vi "CAN Task.vi"(8 "error in":errorcluster, 11 "CANopen Master in":refnum<class "CANopen Master.lvclass">) -> ()   [LabVIEW 2024, in "CANopen Master.lvlib" / "CANopen Master.lvclass"]
uses:
  CANopen Master.lvclass/CANopen Master.ctl
  CANopen Master.lvclass
  CANopen Message/CANopen Message.lvclass
  CANopen Response/CANopen Response Message.lvclass
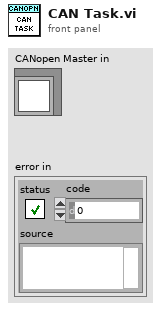
[diagram p1: front panel]
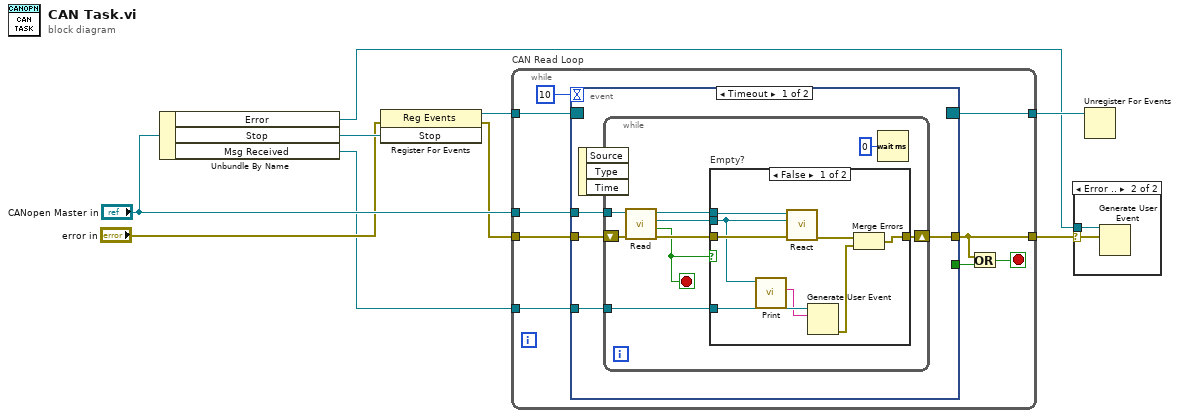
[diagram p0: block diagram]
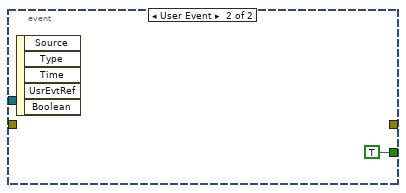
[diagram p4: hidden frame]
diagram:
  n1 = Unbundle By Name("CANopen Master in") -> ("Error"=w1:refnum<user-event>, "Stop"=w6:refnum<user-event>, "Msg Received"=w3:refnum<user-event>)
  n2 = register-events(error in="error in", w6) -> (reference out=w7:refnum<event-registration>, error out=w4:errorcluster)  [unwired: 1 in]
  n3 = while "CAN Read Loop" {
    tunnel: [w14] -> w9
    tunnel: w7 -> [w13]
    tunnel: w3 -> [w11]
    tunnel: "CANopen Master in" -> [w17]
    tunnel: w4 -> [w18]
    tunnel: [w10] -> w2
    stop <- w16 stop-if-true
    n4 = event shown="[0] Timeout" {
      selector: w13 -> [_ _]
      dyn-events: [_ _] -> w14
      timeout: 10 -> [_ _]
      tunnel: w18 -> [w22 _]
      tunnel: w17 -> [w21 _]
      tunnel: [w20 _] -> w10
      tunnel: [_ TRUE] -> w12
      tunnel: w11 -> [w19 _]
      event Timeout {
        n5 = event-data() -> ()  [unwired: 1 in, 3 out]
        n6 = while {
          tunnel: w21 -> [w30]
          tunnel: w19 -> [w28]
          shift-right: [w29] -> w20
          shift-left: w22 -> [w31]
          stop <- w23 stop-if-true
          n7 = call "Read.vi"("error in"=w31, "CANopen Master in"=w30) -> ("error out"=w26:errorcluster, "Empty?"=w23:bool, "CANopen Message out"=w27:refnum<class "CANopen Response Message.lvclass">, "CANopen Master out"=w24:refnum<class "CANopen Master.lvclass">)  [unwired: 6 in]
          n8 = case "Empty?" shown="False" w23 {
            tunnel: w27 -> [w37 _]
            tunnel: [w33 w40] -> w29
            tunnel: w26 -> [w39 w40]
            tunnel: w24 -> [w38 _]
            tunnel: w28 -> [w36 _]
            frame False {
              n9 = call "Print.vi"("CANopen Message in"=w37) -> ("Message"=w35:string)  [unwired: 9 in, 1 out]
              n10 = call "React.vi"("error in"=w39, "CANopen Message"=w37, "CANopen Master in"=w38) -> ("error out"=w34:errorcluster)  [unwired: 7 in, 1 out]
              n11 = Generate User Event(user event=w36, event data cluster=w35) -> (error out=w32:errorcluster)  [unwired: 2 in, 1 out]
              n12 = Merge Errors(w34, w32) -> (w33:errorcluster)
            }
            frame True {
            }
          }
          n13 = Wait (ms)(milliseconds to wait=u32 0) -> ()  [unwired: 1 out]
        }
      }
      event User Event {
        n14 = event-data() -> ()  [unwired: 1 in, 5 out]
      }
    }
    n15 = Or(x=w10, y=w12) -> (x .or. y?=w16:bool)
  }
  n16 = case shown="Error .." w2 {
    selector: w2 -> [_ w42]
    tunnel: w1 -> [_ w43]
    frame No Error {
    }
    frame Error {
      n17 = Generate User Event(user event=w43, event data cluster=w42) -> ()  [unwired: 2 in, 2 out]
    }
  }
  n18 = Unregister For Events(event registration refnum=w9) -> ()  [unwired: 1 in, 1 out]
